vi "Set and Wait to Restart Completion.vi"(8 "error in":errorcluster, 11 "Bool Ref":refnum<vi>) -> (0 "error out":errorcluster)   [LabVIEW 2025, in "CAN-LIN Raw Bus Capture UI.lvlib"]
doc: "Set a bool reference to True and wait till it is set to False.\n\nThis VI not allows completion till the Reference is False again (For example till a restart was done)."
uses:
  CAN-LIN Raw Bus Capture UI.lvlib
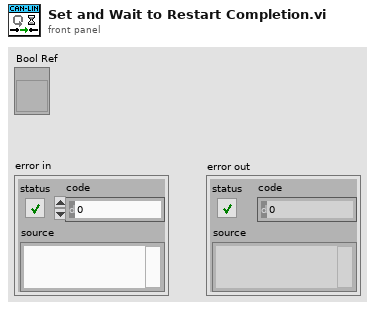
[diagram p1: front panel]
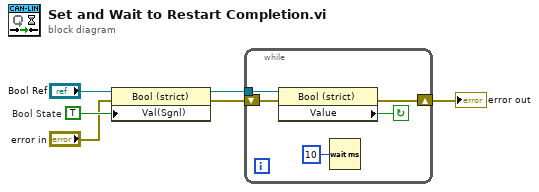
[diagram p0: block diagram]
diagram:
  w6 = TRUE  # Bool State
  n1 = property on="Property Node" class="Bool (strict)"(reference="Bool Ref", error in="error in", "Val(Sgnl)"=w6) -> (reference out=w3:refnum<vi>, error out=w1:errorcluster)
  n2 = while {
    tunnel: w3 -> [w11]
    shift-right: [w8] -> w2
    shift-left: w1 -> [w7]
    stop <- w10 continue-if-true
    n3 = property on="Property Node" class="Bool (strict)"(reference=w11, error in=w7) -> (error out=w8:errorcluster, "Value"=w10:bool)  [unwired: 1 out]
    n4 = Wait (ms)(milliseconds to wait=u32 10) -> ()  [unwired: 1 out]
  }
  "error out" <- w2
